vi "Read Error.vi"(8 "error in (no error)":errorcluster, 11 "GET Async in":refnum<class "GET Async.lvclass">) -> (0 "error out":errorcluster, 2 "error":errorcluster, 3 "GET Async out":refnum<class "GET Async.lvclass">)   [LabVIEW 2019, in "HTTP Client Extensions.lvlib" / "GET Async.lvclass"]
uses:
  GET Async.lvclass
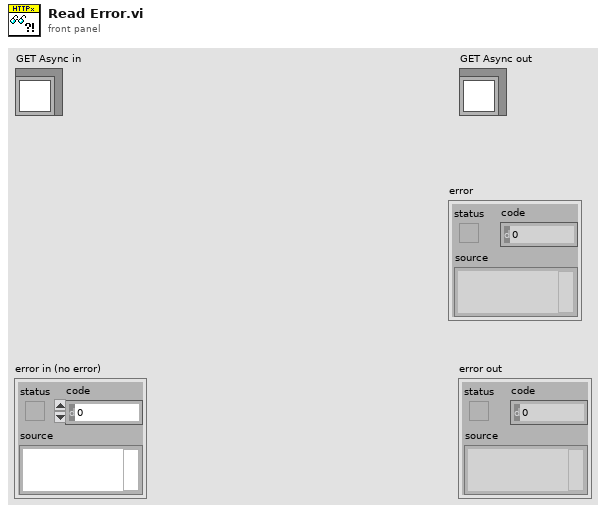
[diagram p1: front panel]
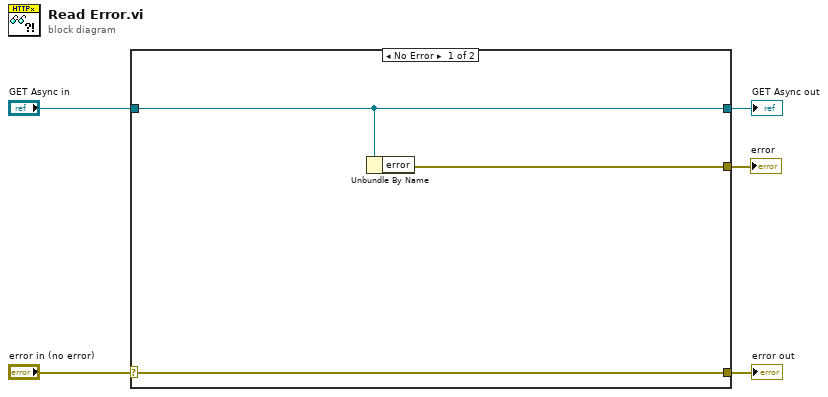
[diagram p0: block diagram]
diagram:
  n1 = case shown="No Error" "error in (no error)" {
    selector: "error in (no error)" -> [w8 w10]
    tunnel: [w8 w10] -> w4
    tunnel: [w7 w9] -> w2
    tunnel: "GET Async in" -> [w7 w9]
    tunnel: [w6 _] -> w1
    frame No Error {
      n2 = Unbundle By Name(w7) -> ("error"=w6:errorcluster)
    }
    frame Error {
    }
  }
  "error out" <- w4
  "GET Async out" <- w2
  "error" <- w1
